vi "Query Questionable Data Register.vi"(8 "error in (no error)":errorcluster, 11 "VISA resource name":refnum<visa-resource-name>) -> (0 "error out":errorcluster, 1 "Questionable Data Message":string, 3 "VISA resource name out":refnum<visa-resource-name>)   [LabVIEW 2014, in "Fluke 884X Series.lvlib"]
doc: "Queries the event register for the Questionable Data Register group. Essentially, it is used to observe possible invalid results. For example, if the set sample interval is less than the minimum sample interval, the questionable data register will be set. This VI will then return the corresponding warning(s)."
uses:
  Fluke 884X Series.lvlib
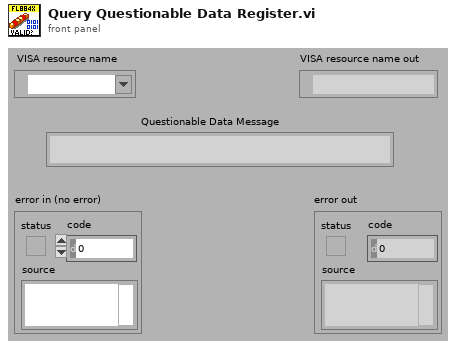
[diagram p1: front panel]
types:
  T1 = cluster{"Boolean array[0]":bool, "Boolean array[1]":bool, "Boolean array[2]":bool, "Boolean array[3]":bool, "Boolean array[4]":bool, "Boolean array[5]":bool, "Boolean array[6]":bool, "Boolean array[7]":bool, "Boolean array[8]":bool, "Boolean array[9]":bool, "Boolean array[10]":bool, "Boolean array[11]":bool, "Boolean array[12]":bool, "Boolean array[13]":bool, "Boolean array[14]":bool, "Boolean array[15]":bool}
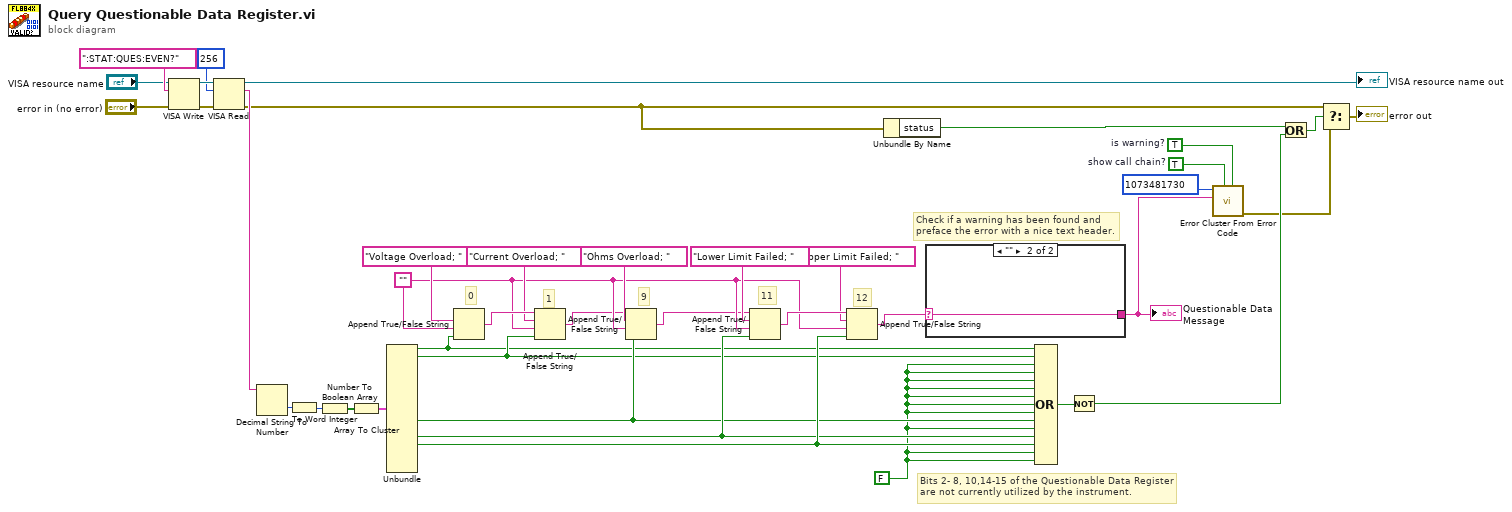
[diagram p0: block diagram]
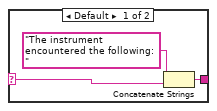
[diagram p2: hidden frame]
diagram:
  w8 = TRUE  # is warning?
  w9 = TRUE  # show call chain?
  w1 = FALSE
  w5 = "" ("Empty String Constant")
  # "12"
  # "11"
  # "9"
  # "1"
  # "0"
  # "Check if a warning has been found and preface the error with a nice text header."
  # "Bits 2- 8, 10,14-15 of the Questionable Data Register are not currently utilized by the instrument."
  n1 = VISA Write(VISA resource name="VISA resource name", write buffer=":STAT:QUES:EVEN?", error in (no error)="error in (no error)") -> (VISA resource name out=w38:refnum<visa-resource-name>, error out=w39:errorcluster)  [unwired: 1 out]
  n2 = VISA Read(VISA resource name=w38, byte count=u32 256, error in (no error)=w39) -> (VISA resource name out=→"VISA resource name out":refnum<visa-resource-name>, read buffer=w36:string, error out=w12:errorcluster)  [unwired: 1 out]
  n3 = Decimal String To Number(string=w36) -> (number=w33:i32)  [unwired: 2 in, 1 out]
  n4 = To Word Integer(number=w33) -> (16bit integer=w34:i16)
  n5 = Number To Boolean Array(number=w34) -> (Boolean array=w35:bool[])
  n6 = Array To Cluster(array=w35) -> (cluster=w32:T1)
  n7 = Unbundle(w32) -> ("Boolean array[0]"=w18:bool, "Boolean array[1]"=w19:bool, "Boolean array[9]"=w20:bool, "Boolean array[11]"=w21:bool, "Boolean array[12]"=w22:bool)  [unwired: 11 out]
  n8 = Append True/False String(1:w18, 2:w5, 3:"Voltage Overload; " ("true string")) -> (0:w31:string)  [unwired: 1 in]
  n9 = Append True/False String(1:w19, 2:w5, 3:"Current Overload; " ("true string"), 4:w31) -> (0:w4:string)
  n10 = Append True/False String(1:w20, 2:w5, 3:"Ohms Overload; " ("true string"), 4:w4) -> (0:w3:string)
  n11 = Append True/False String(1:w21, 2:w5, 3:"Lower Limit Failed; " ("true string"), 4:w3) -> (0:w30:string)
  n12 = Append True/False String(1:w22, 2:w5, 3:"Upper Limit Failed; " ("true string"), 4:w30) -> (0:w2:string)
  n13 = Unbundle By Name(w12) -> ("status"=w15:bool)
  n14 = case shown="\"\"" w2 {
    selector: w2 -> [w42 w44]
    tunnel: [w41 w44] -> w6
    frame Default {
      n15 = Concatenate Strings("The instrument encountered the following: " ("true string"), w42) -> (w41:string)
    }
    frame "" {
    }
  }
  "Questionable Data Message" <- w6
  n16 = Compound Arithmetic op=OR(w18, w19, w1, w1, w1, w1, w1, w1, w1, w20, w1, w21, w22, w1, w1) -> (w17:bool)
  n17 = Not(x=w17) -> (.not. x?=w16:bool)
  n18 = call <vilib>:"Error Cluster From Error Code.vi"("is warning? (False)"=w8, "show call chain? (False)"=w9, "error message (\"\")"=w6, "error code (0)"=1073481730 ("t")) -> ("error out"=w11:errorcluster)  [unwired: 5 in]
  n19 = Or(x=w15, y=w16) -> (x .or. y?=w14:bool)
  n20 = Select(t=w12, s=w14, f=w11) -> (s? t:f=→"error out":errorcluster)
